vi "sub_Image Construct.vi"(10 "Acq.Point":u16[](array[numeric]), 11 "Image Array":dbl[][](array[numeric])) -> (3 "Image Array Out":u16[][](array[numeric]))   [LabVIEW 2015]
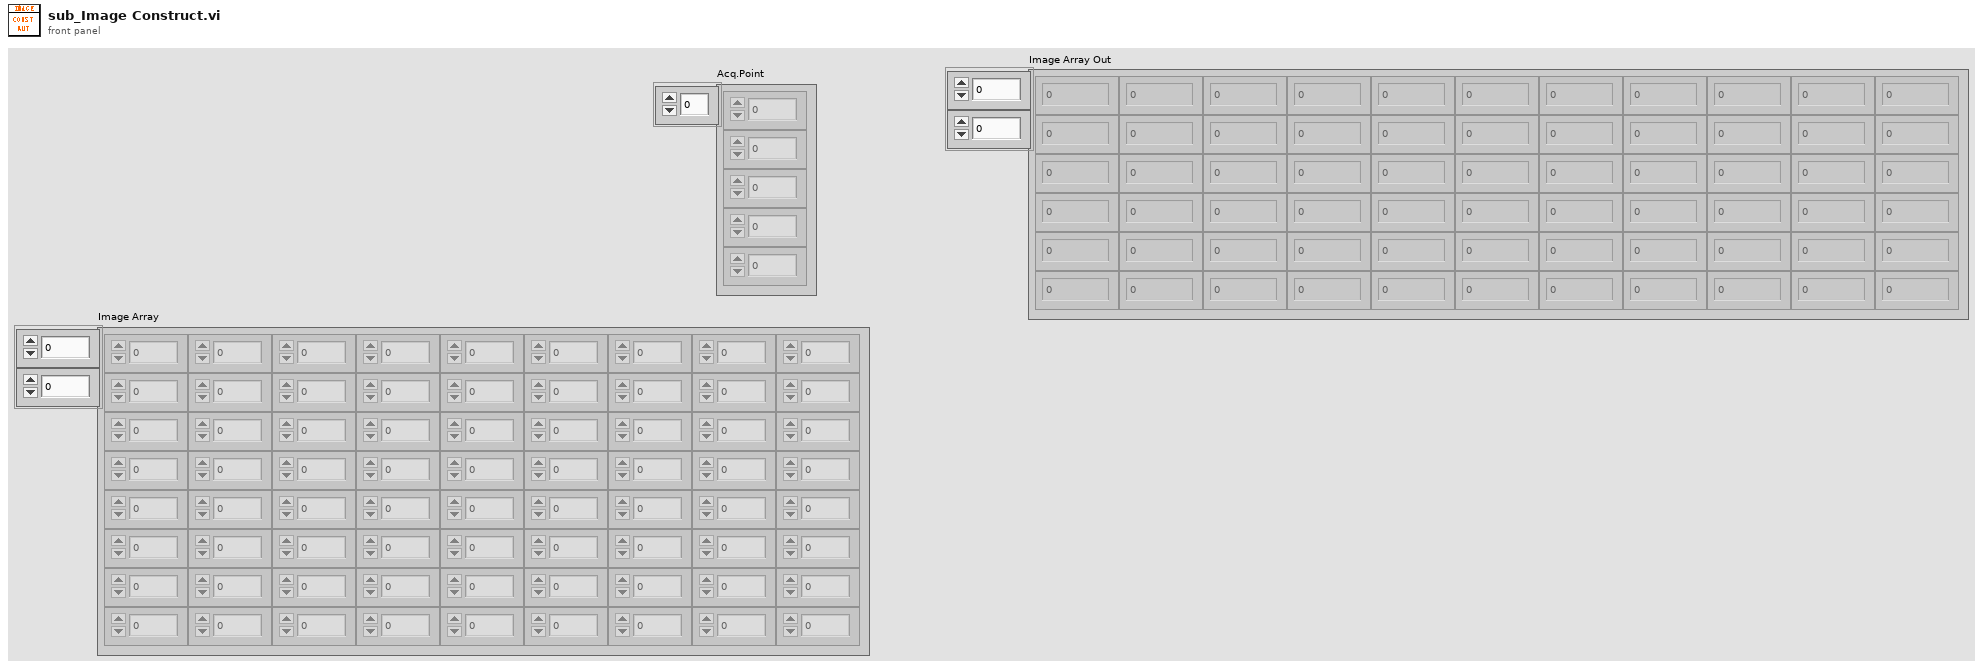
[diagram p1: front panel]
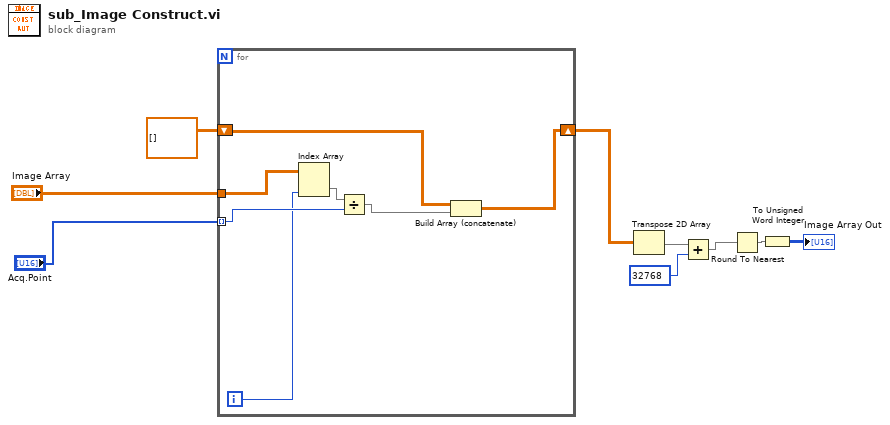
[diagram p0: block diagram]
diagram:
  n1 = for {
    tunnel: "Image Array" -> [w15]
    tunnel: "Acq.Point" -> [w16] mode=indexing
    shift-right: [w10] -> w6
    shift-left: dbl[][] [] -> [w12]
    i -> [w14]
    n2 = Index Array(array=w15, index (col)=w14) -> (element=w13:dbl[])  [unwired: 1 in]
    n3 = Divide(x=w13, y=w16) -> (x/y=w11:dbl[])
    n4 = Build Array (concatenate)(w12, w11) -> (w10:dbl[][])
  }
  n5 = Transpose 2D Array(2D array=w6) -> (transposed array=w3:dbl[][])
  n6 = Add(x=w3, y=32768) -> (x+y=w2:dbl[][])
  n7 = Round To Nearest(number=w2) -> (nearest integer value=w5:dbl[][])
  n8 = To Unsigned Word Integer(number=w5) -> (unsigned 16bit integer=→"Image Array Out":u16[][])
